vi "FormatDMAelement_8_elements_with_scale.vi"(8 "valid in":bool, 10 "factor":u16, 11 "Data in":fxp<+/-,32,14>[](array[numeric])=[0.0, 0.0, 0.0, 0.0, 0.0, 0.0, 0.0, 0.0]) -> (0 "valid out":bool, 3 "Values":u64[](array[numeric]))   [LabVIEW 2018]
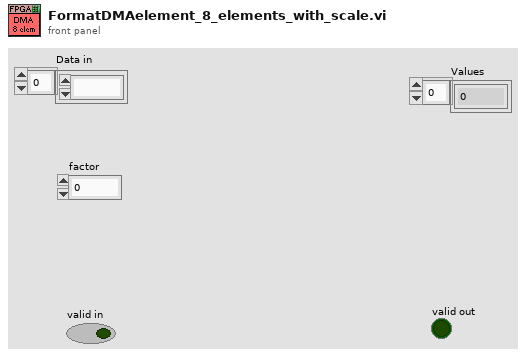
[diagram p1: front panel]
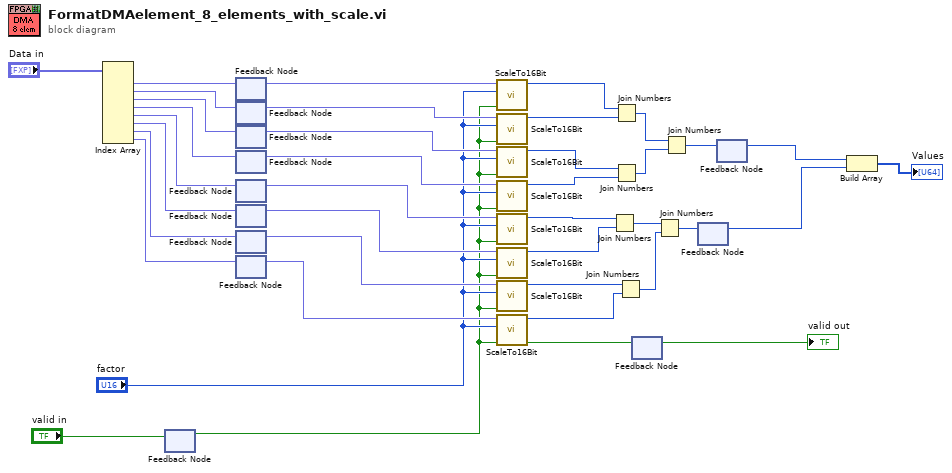
[diagram p0: block diagram]
diagram:
  n1 = Index Array(array="Data in") -> (element #1=w37:fxp<+/-,32,14>, element #2=w36:fxp<+/-,32,14>, element #3=w35:fxp<+/-,32,14>, element #4=w34:fxp<+/-,32,14>, element #5=w31:fxp<+/-,32,14>, element #6=w30:fxp<+/-,32,14>, element #7=w21:fxp<+/-,32,14>, element #8=w20:fxp<+/-,32,14>)  [unwired: 8 in]
  n2 = feedback #1() -> (w10:bool)  [unwired: 1 in]
  n3 = feedback-in #1("valid in") -> ()
  n4 = feedback #2() -> (w19:fxp<+/-,32,14>)  [unwired: 1 in]
  n5 = feedback-in #2(w37) -> ()
  n6 = feedback #3() -> (w18:fxp<+/-,32,14>)  [unwired: 1 in]
  n7 = feedback-in #3(w36) -> ()
  n8 = feedback #4() -> (w17:fxp<+/-,32,14>)  [unwired: 1 in]
  n9 = feedback-in #4(w35) -> ()
  n10 = feedback #5() -> (w16:fxp<+/-,32,14>)  [unwired: 1 in]
  n11 = feedback-in #5(w34) -> ()
  n12 = feedback #6() -> (w15:fxp<+/-,32,14>)  [unwired: 1 in]
  n13 = feedback-in #6(w31) -> ()
  n14 = feedback #7() -> (w14:fxp<+/-,32,14>)  [unwired: 1 in]
  n15 = feedback-in #7(w30) -> ()
  n16 = feedback #8() -> (w13:fxp<+/-,32,14>)  [unwired: 1 in]
  n17 = feedback-in #8(w21) -> ()
  n18 = feedback #9() -> (w12:fxp<+/-,32,14>)  [unwired: 1 in]
  n19 = feedback-in #9(w20) -> ()
  n20 = call "ScaleTo16Bit.vi"("valid in"=w10, "factor"="factor", "Value in"=w19) -> ("16bit integer"=w8:i16)  [unwired: 7 in, 1 out]
  n21 = call "ScaleTo16Bit.vi"("valid in"=w10, "factor"="factor", "Value in"=w18) -> ("16bit integer"=w7:i16)  [unwired: 7 in, 1 out]
  n22 = call "ScaleTo16Bit.vi"("valid in"=w10, "factor"="factor", "Value in"=w17) -> ("16bit integer"=w6:i16)  [unwired: 7 in, 1 out]
  n23 = call "ScaleTo16Bit.vi"("valid in"=w10, "factor"="factor", "Value in"=w16) -> ("16bit integer"=w5:i16)  [unwired: 7 in, 1 out]
  n24 = call "ScaleTo16Bit.vi"("valid in"=w10, "factor"="factor", "Value in"=w15) -> ("16bit integer"=w4:i16)  [unwired: 7 in, 1 out]
  n25 = call "ScaleTo16Bit.vi"("valid in"=w10, "factor"="factor", "Value in"=w14) -> ("16bit integer"=w3:i16)  [unwired: 7 in, 1 out]
  n26 = call "ScaleTo16Bit.vi"("valid in"=w10, "factor"="factor", "Value in"=w13) -> ("16bit integer"=w2:i16)  [unwired: 7 in, 1 out]
  n27 = call "ScaleTo16Bit.vi"("valid in"=w10, "factor"="factor", "Value in"=w12) -> ("valid out"=w9:bool, "16bit integer"=w1:i16)  [unwired: 7 in]
  n28 = Join Numbers(hi=w4, lo=w3) -> ((hi.lo)=w29:u32)
  n29 = Join Numbers(hi=w8, lo=w7) -> ((hi.lo)=w33:u32)
  n30 = Join Numbers(hi=w6, lo=w5) -> ((hi.lo)=w32:u32)
  n31 = Join Numbers(hi=w2, lo=w1) -> ((hi.lo)=w22:u32)
  n32 = feedback #10() -> (→"valid out":bool)  [unwired: 1 in]
  n33 = feedback-in #10(w9) -> ()
  n34 = Join Numbers(hi=w29, lo=w22) -> ((hi.lo)=w27:u64)
  n35 = Join Numbers(hi=w33, lo=w32) -> ((hi.lo)=w28:u64)
  n36 = feedback #11() -> (w26:u64)  [unwired: 1 in]
  n37 = feedback-in #11(w27) -> ()
  n38 = feedback #12() -> (w25:u64)  [unwired: 1 in]
  n39 = feedback-in #12(w28) -> ()
  n40 = Build Array(w25, w26) -> (→"Values":u64[])
